vi "Run Test.vi"(8 "error in (no error)":errorcluster, 11 "Test Template in":refnum<class "Calibration.lvclass">) -> (0 "error out":errorcluster, 1 "Positions":i32[](array[numeric]), 2 "Tests Passed":bool[](array[boolean]), 3 "Test Template out":refnum<class "Calibration.lvclass">, 5 "Fail Codes":string[](array[string]))   [LabVIEW 2015, in "Calibration.lvclass"]
uses:
  Calibration.lvclass
  Test Class/Test Class.lvclass
  Classes/Application/Class/Application.lvclass
  Driver Test/Driver Test.lvclass
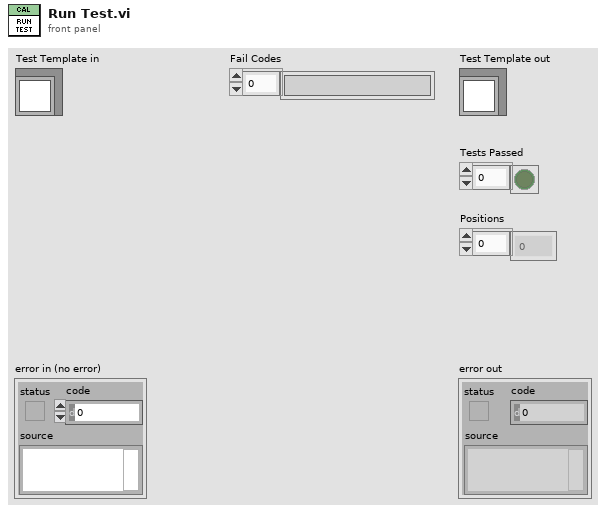
[diagram p1: front panel]
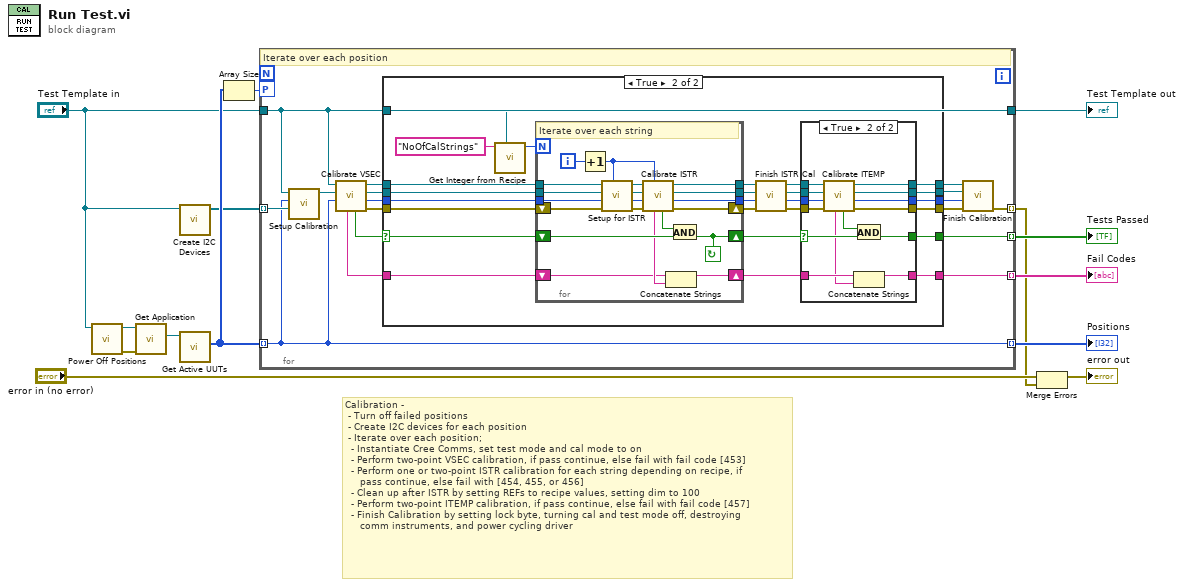
[diagram p0: block diagram]
diagram:
  # "Calibration -\n\t- Turn off failed positions\n\t- Create I2C devices for each position\n\t- Iterate over each position;\n\t\t- Instantiate Cree Comms, set test mode and cal mode to on\n\t\t- Perform two-point VSEC calibration, if pass continue, else fail with fail code [453]\n\t\t- Perform one or two-point ISTR calibration for each string depending on recipe, if \n     pass continue, else fail with [454, 455, or 456]\n\t\t- Clean up after ISTR by setting REFs to recipe values, setting dim to 100\n\t\t- Perform two-point ITEMP calibration, if pass continue, else fail with fail code [457]\n\t\t- Finish Calibration by setting lock byte, turning cal and test mode off, destroying \n     comm instruments, and power cycling driver"
  n1 = call "Power Off Positions.vi"("Driver Test"="Test Template in") -> ("error out"=w9:errorcluster)  [unwired: 10 in]
  n2 = call "Get Application.vi"("error in (no error)"=w9, "Test Class in"="Test Template in") -> ("Application.lvlib:Application.lvclass"=w4:refnum<class "Application.lvclass">)  [unwired: 8 in, 1 out]
  n3 = call "Create I2C Devices.vi"("Driver Test in"="Test Template in") -> ("I2C Devices"=w10:refnum<class "NI-8451.lvclass">[])  [unwired: 9 in, 1 out]
  n4 = call "Get Active UUTs.vi"("Application in"=w4) -> ("Active Positions"=w11:u32[])  [unwired: 8 in, 2 out]
  n5 = Array Size(array=w11) -> (size(s)=w12:i32)
  n6 = for {
    tunnel: w11 -> [w14] mode=indexing
    workers-P: w12 -> [_]
    tunnel: w10 -> [w29] mode=indexing
    tunnel: "Test Template in" -> [w28]
    tunnel: [w28] -> w3
    tunnel: [w22] -> w6 mode=indexing
    tunnel: [w21] -> w8 mode=indexing
    tunnel: [w15] -> w1 mode=indexing
    tunnel: [w14] -> w2 mode=indexing
    # "Iterate over each position"
    n7 = call "Setup Calibration.vi"("Comm Instrument"=w29, "Position"=w14, "Calibration in"=w28) -> ("Cree Communications out"=w30:refnum<class "Cree Communications.lvclass">)  [unwired: 7 in, 1 out]
    n8 = call "Calibrate VSEC.vi"("Position in"=w14, "Cree Comms in"=w30, "Calibration in"=w28) -> ("error out"=w20:errorcluster, "Position out"=w25:u32, "Cree Comms out"=w26:refnum<class "Cree Communications.lvclass">, "Calibration out"=w27:refnum<class "Calibration.lvclass">, "Passed"=w24:bool, "Fail Code"=w23:string)  [unwired: 3 in]
    n9 = case shown="True" w24 {
      selector: w24 -> [w36 w55]
      tunnel: w28 -> [_ w61]
      tunnel: w27 -> [w31 w58]
      tunnel: w26 -> [w33 w57]
      tunnel: w25 -> [w32 w56]
      tunnel: w23 -> [w35 w53]
      tunnel: [w36 w52] -> w22
      tunnel: [w35 w50] -> w21
      tunnel: w20 -> [w34 w49]
      tunnel: [w34 w40] -> w16
      tunnel: [w33 w38] -> w18
      tunnel: [w32 w37] -> w17
      tunnel: [w31 w39] -> w19
      frame False {
      }
      frame True {
        n10 = call "Get Integer from Recipe.vi"("Test Class in"=w61, "Name"="NoOfCalStrings") -> ("Value"=w59:i32)  [unwired: 7 in, 2 out]
        n11 = for {
          N: w59 -> [_]
          tunnel: w58 -> [w91]
          tunnel: w57 -> [w85]
          tunnel: w56 -> [w84]
          shift-right: [w82] -> w54
          shift-left: w55 -> [w95]
          shift-right: [w94] -> w51
          shift-left: w53 -> [w92]
          tunnel: [w100] -> w48
          tunnel: [w99] -> w47
          tunnel: [w98] -> w46
          shift-right: [w97] -> w45
          shift-left: w49 -> [w83]
          i -> [w101]
          stop <- w82 continue-if-true
          # "Iterate over each string"
          n12 = Increment(x=w101) -> (x+1=w89:i32)
          n13 = call "Setup for ISTR.vi"("String"=w89, "error in (no error)"=w83, "Position in"=w84, "Cree Comms in"=w85, "Calibration in"=w91) -> ("error out"=w86:errorcluster, "Position out"=w87:u32, "Cree Comms out"=w88:refnum<class "Cree Communications.lvclass">, "Calibration out"=w90:refnum<class "Calibration.lvclass">)  [unwired: 3 in]
          n14 = call "Calibrate ISTR.vi"("String"=w89, "error in (no error)"=w86, "Position in"=w87, "Cree Comms in"=w88, "Calibration in"=w90) -> ("error out"=w97:errorcluster, "Position out"=w98:u32, "Cree Comms out"=w99:refnum<class "Cree Communications.lvclass">, "Calibration out"=w100:refnum<class "Calibration.lvclass">, "Passed"=w96:bool, "Fail Code"=w93:string)  [unwired: 1 in]
          n15 = Concatenate Strings(w92, w93) -> (w94:string)
          n16 = And(x=w96, y=w95) -> (x .and. y?=w82:bool)
        }
        n17 = call "Finish ISTR Cal.vi"("error in (no error)"=w45, "Position in"=w46, "Cree Comms in"=w47, "Calibration in"=w48) -> ("error out"=w41:errorcluster, "Position out"=w43:u32, "Cree Comms out"=w42:refnum<class "Cree Communications.lvclass">, "Calibration out"=w44:refnum<class "Calibration.lvclass">)  [unwired: 4 in]
        n18 = case shown="True" w54 {
          selector: w54 -> [w67 w81]
          tunnel: [w67 w80] -> w52
          tunnel: w51 -> [w63 w79]
          tunnel: [w63 w78] -> w50
          tunnel: [w66 w77] -> w38
          tunnel: [w65 w76] -> w37
          tunnel: w44 -> [w62 w73]
          tunnel: w43 -> [w65 w72]
          tunnel: w42 -> [w66 w71]
          tunnel: w41 -> [w64 w70]
          tunnel: [w64 w69] -> w40
          tunnel: [w62 w68] -> w39
          frame False {
          }
          frame True {
            n19 = call "Calibrate ITEMP.vi"("error in (no error)"=w70, "Position in"=w72, "Cree Comms in"=w71, "Calibration in"=w73) -> ("error out"=w69:errorcluster, "Position out"=w76:u32, "Cree Comms out"=w77:refnum<class "Cree Communications.lvclass">, "Calibration out"=w68:refnum<class "Calibration.lvclass">, "Passed"=w74:bool, "Fail Code"=w75:string)  [unwired: 2 in]
            n20 = And(x=w74, y=w81) -> (x .and. y?=w80:bool)
            n21 = Concatenate Strings(w79, w75) -> (w78:string)
          }
        }
      }
    }
    n22 = call "Finish Calibration.vi"("Error in"=w16, "Position"=w17, "Cree Comms in"=w18, "Calibration in"=w19) -> ("error out"=w15:errorcluster)  [unwired: 7 in]
  }
  "Test Template out" <- w3
  "Tests Passed" <- w6
  "Fail Codes" <- w8
  "Positions" <- w2
  n23 = Merge Errors("error in (no error)", w1) -> (→"error out":errorcluster)
